vi "MHL Queue Ref Holder.vi"(6 "Action":enum16{"GET", "SET"}(ring), 8 "error in":errorcluster, 11 "Message Queue In":refnum<queue>) -> (0 "error out":errorcluster, 3 "Input Message Queue":refnum<queue>)   [LabVIEW 2015]
doc: "Holds UI queue reference to enqueue messages without wiring"
uses:
  Solution/Production Line/support/Message Queue/Message Cluster.ctl
  Solution/Production Line/support/Message Queue/Message Queue.lvlib
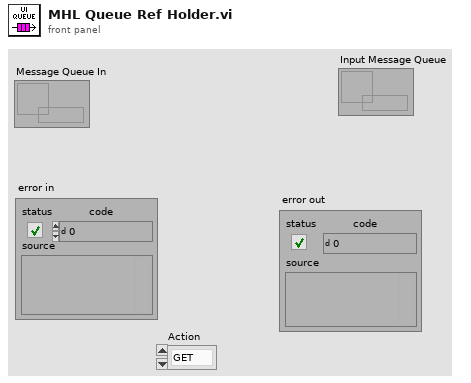
[diagram p1: front panel]
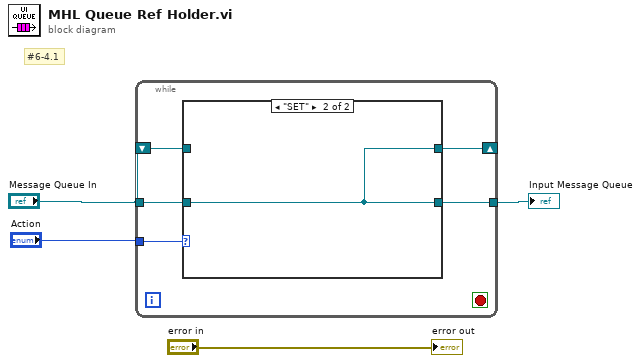
[diagram p0: block diagram]
diagram:
  # "#6-4.1"
  n1 = while {
    tunnel: "Message Queue In" -> [w8]
    tunnel: [w5] -> w4
    tunnel: "Action" -> [w9]
    shift-right: [w6] -> _
    shift-left: "Message Queue In" -> [w7]
    stop <- _ stop-if-true
    n2 = case shown="\"SET\"" w9 {
      tunnel: w8 -> [_ w11]
      tunnel: [w10 w11] -> w6
      tunnel: w7 -> [w10 _]
      tunnel: [w10 w11] -> w5
      frame "GET", Default {
      }
      frame "SET" {
      }
    }
  }
  "Input Message Queue" <- w4
  "error out" <- "error in"
